vi "Evaluate Hall Test 1.vi"(1 "String In":string) -> (0 "Test OK":bool)   [LabVIEW 2023]
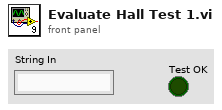
[diagram p1: front panel]
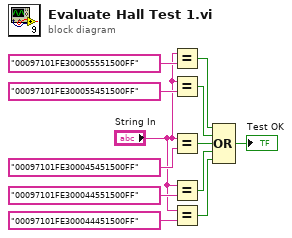
[diagram p0: block diagram]
diagram:
  n1 = Equal?(x="String In", y="00097101FE300055551500FF" ("Self Test BIST")) -> (x = y?=w8:bool)
  n2 = Equal?(x="String In", y="00097101FE300055451500FF") -> (x = y?=w7:bool)
  n3 = Equal?(x="String In", y="00097101FE300045451500FF") -> (x = y?=w6:bool)
  n4 = Equal?(x="String In", y="00097101FE300044551500FF") -> (x = y?=w5:bool)
  n5 = Equal?(x="String In", y="00097101FE300044451500FF") -> (x = y?=w1:bool)
  n6 = Compound Arithmetic op=OR(w8, w7, w6, w5, w1) -> (→"Test OK":bool)
